vi "Pullability.vi"(0 "Power Supply Address":u8=5, 1 "PowerSupplyType":i32, 3 "Output Terminals(+6 V:0)":u16(ring) items=["+6 V output", "+25 V output", "-25 V output"], 4 "Frequency Counter Address":i16=3 max=31, 5 "Frequency Channel":enum16{"Channel 1", "Channel 2", "Channel 3"}(ring), 6 "Gate Time":T1(ring)=enum."1.0 second", 7 "Ideal V_inj":dbl format="%.4f") -> (2 "Pullability":dbl format="%.6f")   [LabVIEW 2024]
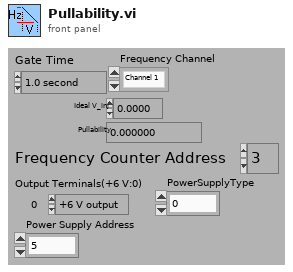
[diagram p1: front panel]
types:
  T1 = enum16{"0.1 second", "1.0 second", "10.0 second"}
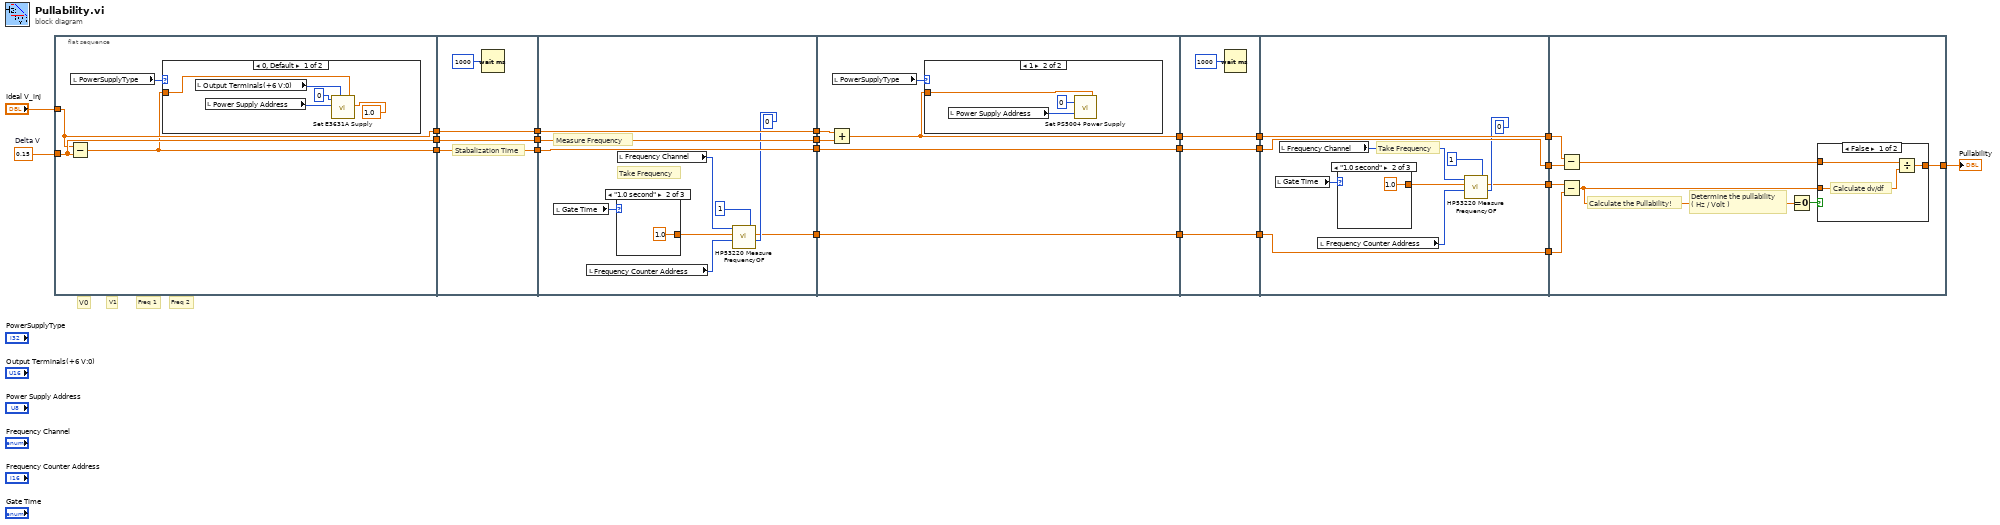
[diagram p0: block diagram]
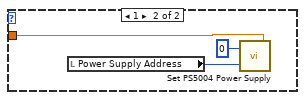
[diagram p2: hidden frame]
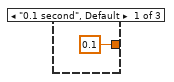
[diagram p3: hidden frame]
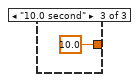
[diagram p4: hidden frame]
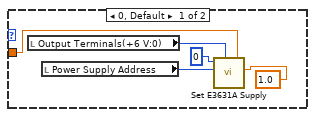
[diagram p5: hidden frame]
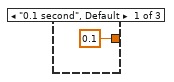
[diagram p6: hidden frame]
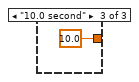
[diagram p7: hidden frame]
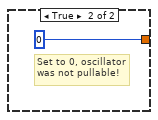
[diagram p8: hidden frame]
diagram:
  w22 = 0.15  # Delta V
  # "V1"
  # "V0"
  # "Freq 2"
  # "Freq 1"
  n1 = flat-sequence {
    tunnel: "Ideal V_inj" -> [w26]
    tunnel: [w26] -> w20
    tunnel: w22 -> [w27]
    tunnel: [w27] -> w19
    tunnel: [w24] -> w18
    tunnel: w20 -> [w38]
    tunnel: [w38] -> w17
    tunnel: w19 -> [w37]
    tunnel: [w37] -> w16
    tunnel: w18 -> [w36]
    tunnel: [w36] -> w15
    tunnel: w17 -> [w49]
    tunnel: [w49] -> w14
    tunnel: w16 -> [w48]
    tunnel: [w48] -> w13
    tunnel: [w40] -> w12
    tunnel: w15 -> [w47]
    tunnel: [w47] -> w11
    tunnel: w14 -> [w58]
    tunnel: w13 -> [w57]
    tunnel: w12 -> [w56]
    tunnel: [w56] -> w10
    tunnel: w11 -> [w55]
    tunnel: [w55] -> w9
    tunnel: [w53] -> w8
    tunnel: w10 -> [w69]
    tunnel: [w69] -> w7
    tunnel: w9 -> [w68]
    tunnel: [w68] -> w6
    tunnel: w8 -> [w67]
    tunnel: [w67] -> w5
    tunnel: [w71] -> w4
    tunnel: w7 -> [w80]
    tunnel: [w80] -> w3
    tunnel: w6 -> [w79]
    tunnel: [w79] -> w2
    tunnel: w5 -> [w78]
    tunnel: [w78] -> w1
    tunnel: [w84] -> w21
    tunnel: w4 -> [w91]
    tunnel: w3 -> [w90]
    tunnel: w2 -> [w88]
    tunnel: w1 -> [w89]
    frame #0 {
      n2 = Subtract(x=w26, y=w27) -> (x-y=w24:dbl)
      n3 = local read "PowerSupplyType"() -> (w25:i32)
      n4 = case shown="0, Default" w25 {
        tunnel: w24 -> [w32 w34]
        frame 0, Default {
          n5 = local read "Output Terminals(+6 V:0)"() -> (w29:u16)
          n6 = local read "Power Supply Address"() -> (w30:u8)
          n7 = call "Set E3631A Supply.vi"("Current Limit"=1.0, "Voltage Limit"=w32, "Output Terminals(+6 V:0)"=w29, "Address"=w30, "GPIB#"=u8 0) -> ()  [unwired: 3 in, 1 out]
        }
        frame 1 {
          n8 = local read "Power Supply Address"() -> (w33:u8)
          n9 = call "Set PS5004 Power Supply.vi"("Voltage"=w34, "Address"=w33, "System#"=0) -> ()
        }
      }
    }
    frame #1 {
      # "Stabalization Time"
      n10 = Wait (ms)(milliseconds to wait=u32 1000) -> ()  [unwired: 1 out]
    }
    frame #2 {
      # "Take Frequency"
      # "Measure Frequency"
      n11 = local read "Gate Time"() -> (w46:T1)
      n12 = local read "Frequency Counter Address"() -> (w44:i16)
      n13 = case shown="\"1.0 second\"" w46 {
        tunnel: [0.1 ("Gate Time") 1.0 ("Gate Time") 10.0 ("Gate Time")] -> w45
        frame "0.1 second", Default {
        }
        frame "1.0 second" {
        }
        frame "10.0 second" {
        }
      }
      n14 = local read "Frequency Channel"() -> (w41:enum16{"Channel 1", "Channel 2", "Channel 3"})
      n15 = call "HP53220 Measure FrequencyOF.vi"("GPIB Bus"=0, "Number of Readings"=1, "GPIB Address"=w44, "Gate Time"=w45, "Channel(1,2,3)"=w41) -> ("Frequency"=w40:dbl)  [unwired: 1 in, 1 out]
    }
    frame #3 {
      n16 = Add(x=w58, y=w57) -> (x+y=w53:dbl)
      n17 = local read "PowerSupplyType"() -> (w54:i32)
      n18 = case shown="1" w54 {
        tunnel: w53 -> [w63 w65]
        frame 0, Default {
          n19 = local read "Output Terminals(+6 V:0)"() -> (w60:u16)
          n20 = local read "Power Supply Address"() -> (w61:u8)
          n21 = call "Set E3631A Supply.vi"("Current Limit"=1.0, "Voltage Limit"=w63, "Output Terminals(+6 V:0)"=w60, "Address"=w61, "GPIB#"=u8 0) -> ()  [unwired: 3 in, 1 out]
        }
        frame 1 {
          n22 = local read "Power Supply Address"() -> (w64:u8)
          n23 = call "Set PS5004 Power Supply.vi"("Voltage"=w65, "Address"=w64, "System#"=0) -> ()
        }
      }
    }
    frame #4 {
      n24 = Wait (ms)(milliseconds to wait=u32 1000) -> ()  [unwired: 1 out]
    }
    frame #5 {
      # "Take Frequency"
      n25 = local read "Gate Time"() -> (w77:T1)
      n26 = local read "Frequency Channel"() -> (w72:enum16{"Channel 1", "Channel 2", "Channel 3"})
      n27 = local read "Frequency Counter Address"() -> (w75:i16)
      n28 = case shown="\"1.0 second\"" w77 {
        tunnel: [0.1 ("Gate Time") 1.0 ("Gate Time") 10.0 ("Gate Time")] -> w76
        frame "0.1 second", Default {
        }
        frame "1.0 second" {
        }
        frame "10.0 second" {
        }
      }
      n29 = call "HP53220 Measure FrequencyOF.vi"("GPIB Bus"=0, "Number of Readings"=1, "GPIB Address"=w75, "Gate Time"=w76, "Channel(1,2,3)"=w72) -> ("Frequency"=w71:dbl)  [unwired: 1 in, 1 out]
    }
    frame #6 {
      # "Determine the pullability\n( Hz / Volt )"
      # "Calculate the Pullability!"
      n30 = Subtract(x=w89, y=w88) -> (x-y=w85:dbl)
      n31 = Subtract(x=w91, y=w90) -> (x-y=w86:dbl)
      n32 = Equal To 0?(x=w86) -> (x = 0?=w87:bool)
      n33 = case shown="False" w87 {
        tunnel: w86 -> [w94 _]
        tunnel: w85 -> [w93 _]
        tunnel: [w92 0] -> w84
        frame False {
          # "Calculate dv/df"
          n34 = Divide(x=w93, y=w94) -> (x/y=w92:dbl)
        }
        frame True {
          # "Set to 0, oscillator\nwas not pullable!"
        }
      }
    }
  }
  "Pullability" <- w21
